vi "5.0-Functional Global for Act Neurons.vi"(1 "Input Act Neurons":T1, 2 "Mode":enum16{"Set Hypothalamus", "Read Hypothalamus"}(ring)=enum."Read Hypothalamus") -> (0 "Output Act Neurons":T1)   [LabVIEW 2010]
uses:
  4-High Neurons/4.1.2-Act Neuron TD.ctl
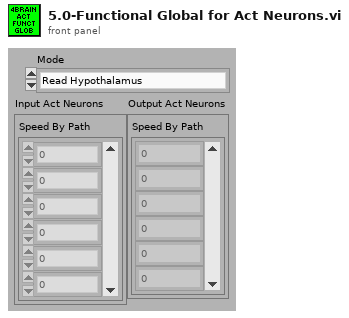
[diagram p1: front panel]
types:
  T1 = typedef "4.1.2-Act Neuron TD.ctl" = cluster{"Speed By Path":sgl[]}
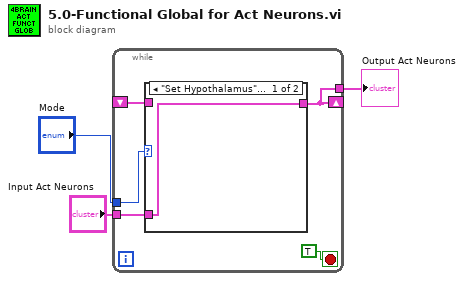
[diagram p0: block diagram]
diagram:
  n1 = while {
    shift-right: [w5] -> _
    shift-left: _ -> [w6]
    tunnel: "Mode" -> [w7]
    tunnel: "Input Act Neurons" -> [w4]
    tunnel: [w5] -> w1
    stop <- TRUE stop-if-true
    n2 = case shown="\"Set Hypothalamus\", Default" w7 {
      tunnel: [w9 w10] -> w5
      tunnel: w6 -> [_ w10]
      tunnel: w4 -> [w9 _]
      frame "Set Hypothalamus", Default {
      }
      frame "Read Hypothalamus" {
      }
    }
  }
  "Output Act Neurons" <- w1
